vi "Calc_Parallel_Throw_Resitance_any num throws.vi"(11 "Resitance_Per Site":dbl[](array[numeric])) -> (3 "Parallel_Resitance":dbl[](array[numeric]))   [LabVIEW 2013]
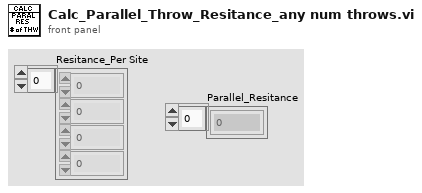
[diagram p1: front panel]
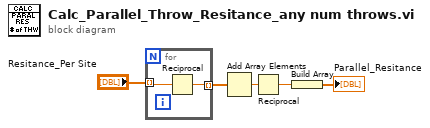
[diagram p0: block diagram]
diagram:
  n1 = for {
    tunnel: "Resitance_Per Site" -> [w7] mode=indexing
    tunnel: [w6] -> w5 mode=indexing
    n2 = Reciprocal(x=w7) -> (1/x=w6:dbl)
  }
  n3 = Add Array Elements(numeric array=w5) -> (sum=w4:dbl)
  n4 = Reciprocal(x=w4) -> (1/x=w2:dbl)
  n5 = Build Array(w2) -> (→"Parallel_Resitance":dbl[])
